vi "OpenSP.vi"(8 "error in (no error)":errorcluster, 10 "path to db simulation":path, 11 "SimulationParameter in":refnum<class "SimulationParameter.lvclass">) -> (0 "error out":errorcluster, 3 "SimulationParameter out":refnum<class "SimulationParameter.lvclass">)   [LabVIEW 2017, in "SimulationParameter.lvclass"]
uses:
  SimulationParameter.lvclass
  SimulationParameter.lvclass/SimulationParameter.ctl
  <vilib>/drjdpowell/SQLite Library/SQL Connection/Open (path).vi
  <vilib>/drjdpowell/SQLite Library/SQL Connection/Open (string).vi
  <vilib>/AdvancedString/Path To Command Line String.vi
  <vilib>/drjdpowell/SQLite Library/SQL Connection/Connection.lvclass
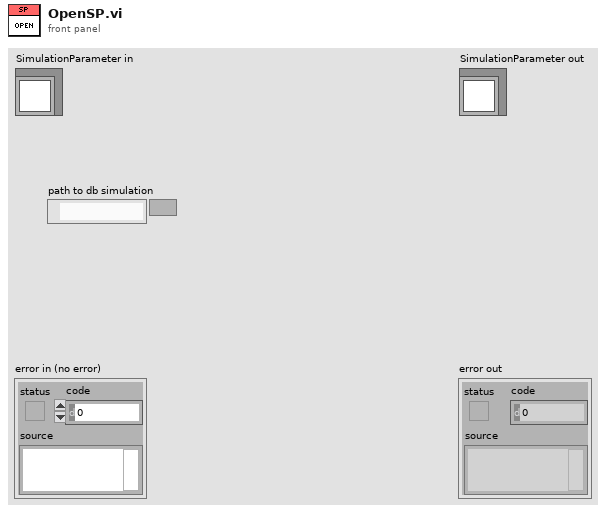
[diagram p1: front panel]
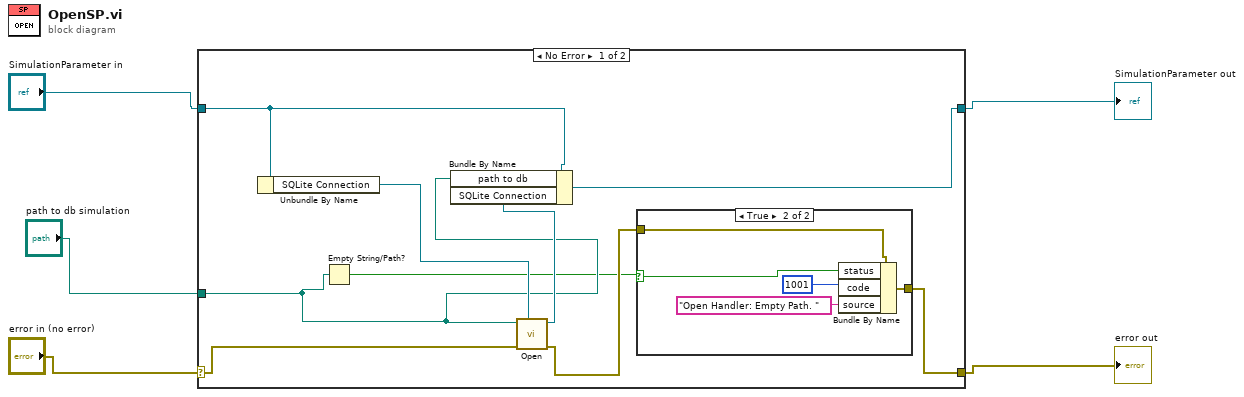
[diagram p0: block diagram]
diagram:
  n1 = case shown="No Error" "error in (no error)" {
    selector: "error in (no error)" -> [w14 w21]
    tunnel: [w8 w21] -> w3
    tunnel: [w13 w22] -> w2
    tunnel: "SimulationParameter in" -> [w12 w22]
    tunnel: "path to db simulation" -> [w7 _]
    frame No Error {
      n2 = Unbundle By Name(w12) -> ("SQLite Connection"=w11:refnum<class "Connection.lvclass">)
      n3 = Empty String/Path?(string/path=w7) -> (empty?=w6:bool)
      n4 = call-poly <vilib>:"Open.vi"("SQLite Connection type"=w11, "error in (no error)"=w14, "db file"=w7) -> ("error out"=w9:errorcluster, "SQLite Connection out"=w10:refnum<class "Connection.lvclass">)  [unwired: 7 in]
      n5 = Bundle By Name(cluster=w12, "path to db"=w7, "SQLite Connection"=w10) -> (w13:refnum<class "SimulationParameter.lvclass">)
      n6 = case shown="True" w6 {
        selector: w6 -> [_ w16]
        tunnel: w9 -> [w15 w18]
        tunnel: [w15 w17] -> w8
        frame False {
        }
        frame True {
          n7 = Bundle By Name(cluster=w18, "status"=w16, "code"=1001, "source"="Open Handler: Empty Path. ") -> (w17:errorcluster)
        }
      }
    }
    frame Error {
    }
  }
  "error out" <- w3
  "SimulationParameter out" <- w2
